vi "Shared Variable Container Filename and Path--Const.vi"() -> (3 "Path to Shared Variable Containing Library":path)   [LabVIEW 2017, in "Shared Variables Library.lvlib"]
doc: "Path to the library, where the shared variables will be stored and deployed from."
uses:
  Shared Variables Library.lvlib
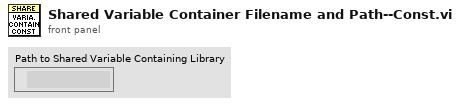
[diagram p1: front panel]
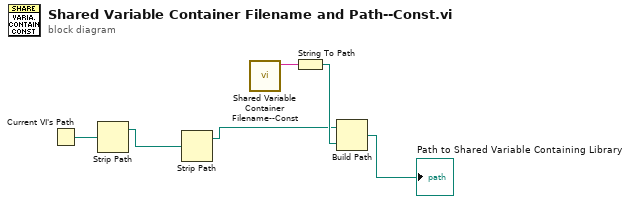
[diagram p0: block diagram]
diagram:
  n1 = Current VI's Path() -> (path=w3:path)
  n2 = Strip Path(path=w3) -> (stripped path=w2:path)  [unwired: 1 out]
  n3 = Strip Path(path=w2) -> (stripped path=w1:path)  [unwired: 1 out]
  n4 = call "Shared Variable Container Filename--Const.vi"() -> ("Shared Variables Container Filename"=w4:string)  [unwired: 11 in]
  n5 = String To Path(string=w4) -> (path=w5:path)
  n6 = Build Path(base path=w1, name or relative path=w5) -> (appended path=→"Path to Shared Variable Containing Library":path)
